vi "Begin.vi"(8 "error in":errorcluster) -> (0 "error out":errorcluster)   [LabVIEW 2019]
doc: "Called before other user functions, this VI is expected to open initial I/O refnums, load in file data, and do all program initialization. Notice that the <B>error out</B> terminal is simply used for data flow. Wiring it to other structures or subVIs ensures that this VI runs first."
uses:
  Robot Global Data.vi
  <vilib>/Rock Robotics/WPI/DriverStation/WPI_DriverStationRobotMode2.ctl
  <vilib>/Rock Robotics/WPI/Joystick/WPI_JoystickDeviceEnum.ctl
  <vilib>/Rock Robotics/Network Tables/NT Write String Array.vi
  <vilib>/Rock Robotics/WPI/ThirdParty/Phoenix-LabVIEW/Motor Controller/Controls/CTRE_Phoenix_MotorControl_NeutralMode.ctl
  <vilib>/Rock Robotics/WPI/SafetyOutput/WPI_SafetyOutputConfigMenu.ctl
  <vilib>/Rock Robotics/WPI/ThirdParty/Phoenix-LabVIEW/Motor Controller/Controls/CTRE_Phoenix_MotorControl_StatusFrameEnhanced.ctl
  <vilib>/Rock Robotics/WPI/ThirdParty/Phoenix-LabVIEW/Motor Controller/Controls/CTRE_Phoenix_MotorControl_ControlMode.ctl
  <vilib>/Rock Robotics/WPI/ThirdParty/Phoenix-LabVIEW/Motor Controller/Controls/CTRE_Phoenix_MotorControl_FeedbackDevice_TalonFX.ctl
  <vilib>/Rock Robotics/WPI/ThirdParty/Phoenix-LabVIEW/CANCoder/Controls/CTRE_Phoenix_CANcoder_SensorInitializationStrategy.ctl
  <vilib>/Rock Robotics/WPI/ThirdParty/Phoenix-LabVIEW/Motor Controller/Sensor/CTRE_Phoenix_MotorControl_SetIntegratedSensorPosition_TalonFX.vi
  <vilib>/Rock Robotics/WPI/RobotDrive/WPI_RobotDriveOpen4MotorWithExistingMotors.vi
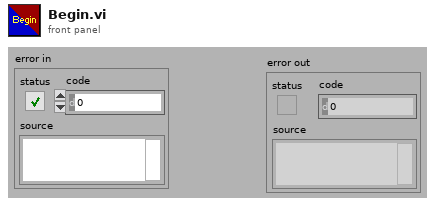
[diagram p1: front panel]
types:
  T1 = typedef "CTRE_Phoenix_MotorControl_NeutralMode.ctl" = enum8{"EEPROMSetting", "Override to Coast", "Override to Brake"}
  T2 = typedef "CTRE_Phoenix_MotorControl_ControlMode.ctl" = u16
  T3 = typedef "CTRE_Phoenix_MotorControl_StatusFrameEnhanced.ctl" = u16
  T4 = typedef "WPI_SafetyOutputConfigMenu.ctl" = enum16{"Enable", "Disable"}
  T5 = typedef "CTRE_Phoenix_CANcoder_SensorInitializationStrategy.ctl" = enum16{"Boot To Zero", "Boot To Absolute Position"}
  T6 = typedef "CTRE_Phoenix_MotorControl_FeedbackDevice_TalonFX.ctl" = i8
  T7 = typedef "WPI_JoystickDeviceEnum.ctl" = enum16{"USB 0", "USB 1", "USB 2", "USB 3", "USB 4", "USB 5"}
  T8 = typedef "WPI_DriverStationRobotMode2.ctl" = enum16{"Autonomous Disabled", "Autonomous Enabled", "Teleop Disabled", "Teleop Enabled", "Disconnected", "Finish", "Test Disabled", "Test Enabled", "Emergency Stopped"}
  T9 = typedef "WPI_JoystickDevRef.ctl" = cluster{"Device":T7}
  T10 = typedef "WPI_MotorControlDeviceRef.ctl" = cluster{"DeviceStatus":errorcluster, "Type":T11, "PWM":cluster{"PWM Channel":T12, "DeadBand":T13}, "CAN":cluster{"Device Number":u8, "SetOutput VI Ref":variant, "GetOutput VI Ref":variant, "Enable VI Ref":variant, "Disable VI Ref":variant, "Data":variant}, "Invert":bool, "DIO PWM":cluster{"PWM \"Enable\" Channel":T12, "DIOChannel":T14, "PWM Rate":dbl}}
  T11 = typedef "WPI_MotorControlType.ctl" = enum16{"PWM", "CAN", "DIO PWM"}
  T12 = typedef "FPGA_DIOPWMChannel.ctl" = enum8{"PWM 0", "PWM 1", "PWM 2", "PWM 3", "PWM 4", "PWM 5", "PWM 6", "PWM 7", "PWM 8", "PWM 9", "PWM MXP 0", "PWM MXP 1", "PWM MXP 2", "PWM MXP 3", "PWM MXP 4", "PWM MXP 5", "PWM MXP 6", "PWM MXP 7", "PWM MXP 8", "PWM MXP 9", "Invalid"}
  T13 = typedef "WPI_PWMDeadband.ctl" = cluster{"Name":string, "maxPositivePwm":i32, "minPositivePwm":i32, "centerPwm":i32, "maxNegativePwm":i32, "minNegativePwm":i32, "angularRange":u16}
  T14 = typedef "FPGA_DIOChannel.ctl" = enum8{"DIO 0", "DIO 1", "DIO 2", "DIO 3", "DIO 4", "DIO 5", "DIO 6", "DIO 7", "DIO 8", "DIO 9", "DIO MXP 0", "DIO MXP 1", "DIO MXP 2", "DIO MXP 3", "DIO MXP 4", "DIO MXP 5", "DIO MXP 6", "DIO MXP 7", "DIO MXP 8", "DIO MXP 9", "DIO MXP 10", "DIO MXP 11", "DIO MXP 12", "DIO MXP 13", "DIO MXP 14", "DIO MXP 15", "SPI Port CS1", "SPI Port CS2", "SPI Port CS3", "SPI Port MISO", "SPI Port MOSI", "Invalid"}
  T15 = typedef "WPI_RobotDriveDevRef.ctl" = cluster{"DevStatus":errorcluster, "Motors[]":T10[], "Square Inputs":bool, "Max Output":dbl}
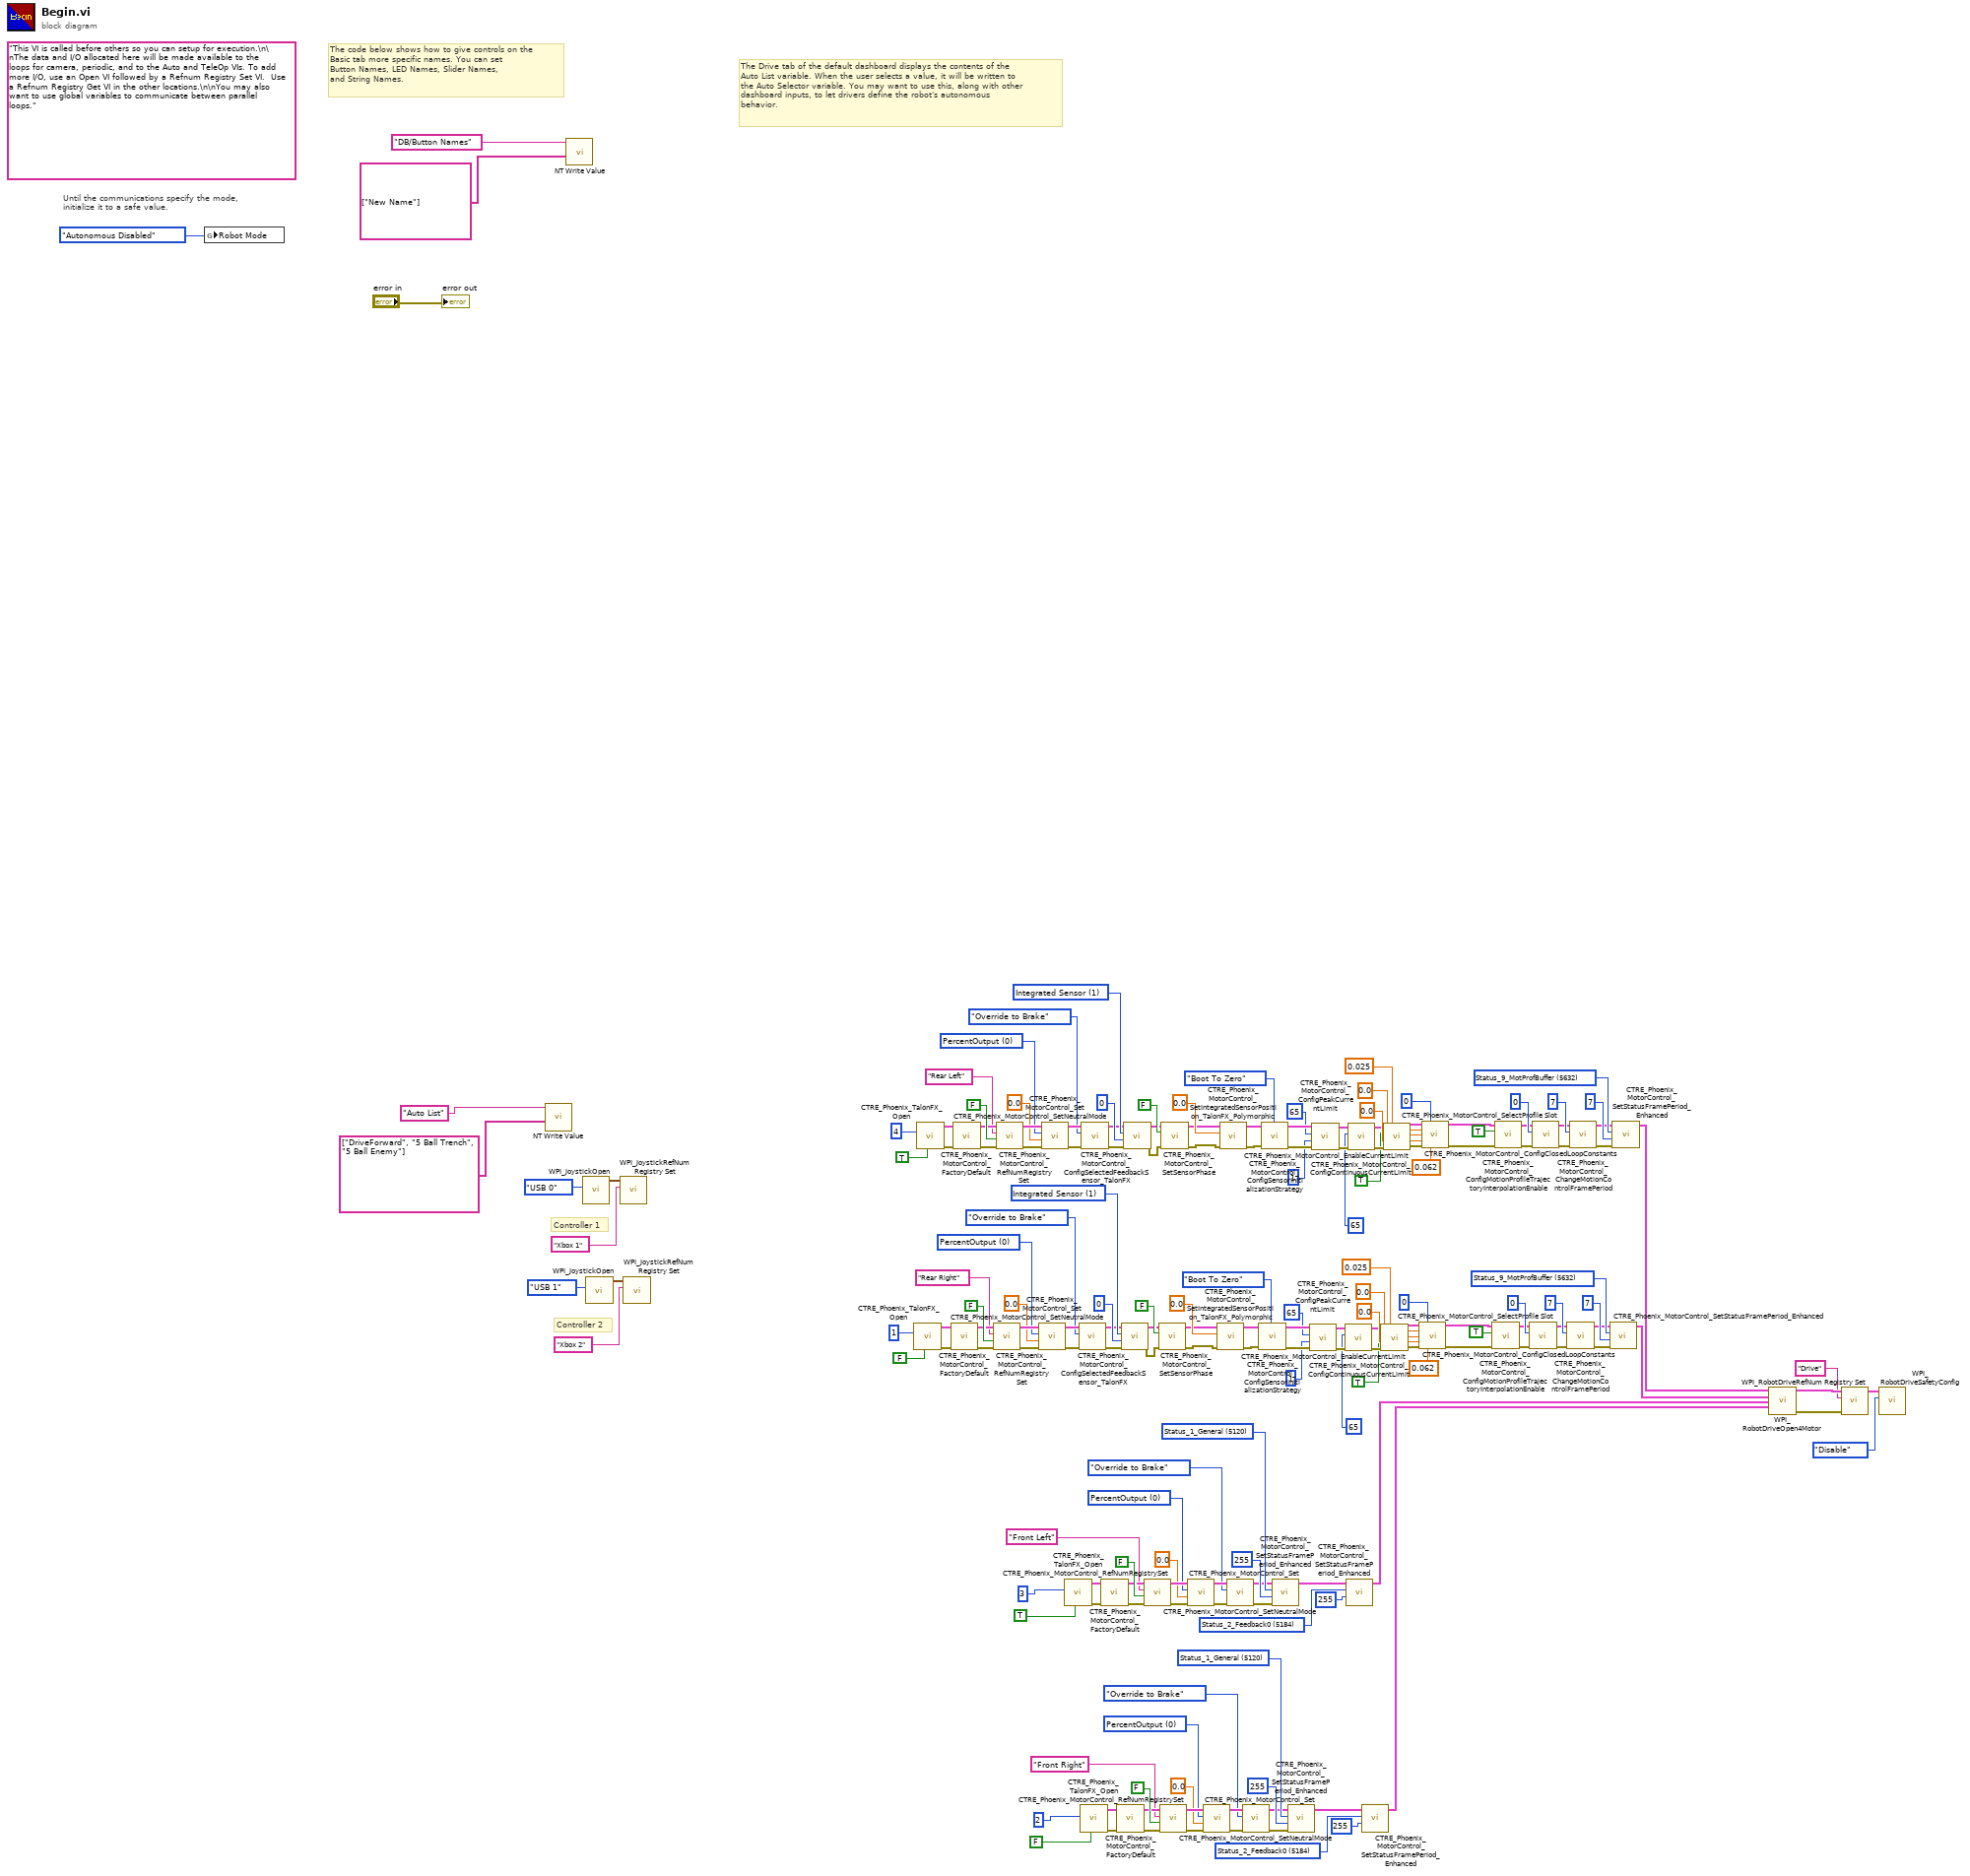
[diagram p0: block diagram]
diagram:
  w14 = T2 0 items=["PercentOutput"=0, "Position"=1, "Velocity"=2, "Current"=3, "Follower"=5, "MotionProfile"=6, "MotionMagic"=7, "MotionProfileArc"=10, "Disabled"=15] ("Control Mode")
  w21 = T3 5184 items=["Status_1_General"=5120, "Status_2_Feedback0"=5184, "Status_3_Quadrature"=5248, "Status_4_AinTempVbat"=5312, "Status_6_Misc"=5440, "Status_7_CommStatus"=5504, "Status_8_PulseWidth"=5568, "Status_9_MotProfBuffer"=5632, "Status_10_MotionMagic"=5696, "Status_11_UartGadgeteer"=5760, "Status_12_Feedback1"=5824, "Status_13_Base_PIDF0"=5888, "Status_14_Turn_PIDF1"=5952, "Status_15_FirmwareApiStatus"=6016] ("Status Frame")
  w23 = T3 5120 items=["Status_1_General"=5120, "Status_2_Feedback0"=5184, "Status_3_Quadrature"=5248, "Status_4_AinTempVbat"=5312, "Status_6_Misc"=5440, "Status_7_CommStatus"=5504, "Status_8_PulseWidth"=5568, "Status_9_MotProfBuffer"=5632, "Status_10_MotionMagic"=5696, "Status_11_UartGadgeteer"=5760, "Status_12_Feedback1"=5824, "Status_13_Base_PIDF0"=5888, "Status_14_Turn_PIDF1"=5952, "Status_15_FirmwareApiStatus"=6016] ("Status Frame")
  w37 = T2 0 items=["PercentOutput"=0, "Position"=1, "Velocity"=2, "Current"=3, "Follower"=5, "MotionProfile"=6, "MotionMagic"=7, "MotionProfileArc"=10, "Disabled"=15] ("Control Mode")
  w44 = T3 5184 items=["Status_1_General"=5120, "Status_2_Feedback0"=5184, "Status_3_Quadrature"=5248, "Status_4_AinTempVbat"=5312, "Status_6_Misc"=5440, "Status_7_CommStatus"=5504, "Status_8_PulseWidth"=5568, "Status_9_MotProfBuffer"=5632, "Status_10_MotionMagic"=5696, "Status_11_UartGadgeteer"=5760, "Status_12_Feedback1"=5824, "Status_13_Base_PIDF0"=5888, "Status_14_Turn_PIDF1"=5952, "Status_15_FirmwareApiStatus"=6016] ("Status Frame")
  w46 = T3 5120 items=["Status_1_General"=5120, "Status_2_Feedback0"=5184, "Status_3_Quadrature"=5248, "Status_4_AinTempVbat"=5312, "Status_6_Misc"=5440, "Status_7_CommStatus"=5504, "Status_8_PulseWidth"=5568, "Status_9_MotProfBuffer"=5632, "Status_10_MotionMagic"=5696, "Status_11_UartGadgeteer"=5760, "Status_12_Feedback1"=5824, "Status_13_Base_PIDF0"=5888, "Status_14_Turn_PIDF1"=5952, "Status_15_FirmwareApiStatus"=6016] ("Status Frame")
  w94 = T6 1 items=["Integrated Sensor"=1, "Sensor Sum (S0 + S1)"=9, "Sensor Difference (D0 - D1)"=10, "Remote Source 0"=11, "Remote Source 1"=12, "None"=14, "Software Emulated"=15] ("Talon FX Feedback Device")
  w96 = T2 0 items=["PercentOutput"=0, "Position"=1, "Velocity"=2, "Current"=3, "Follower"=5, "MotionProfile"=6, "MotionMagic"=7, "MotionProfileArc"=10, "Disabled"=15] ("Control Mode")
  w111 = T3 5632 items=["Status_1_General"=5120, "Status_2_Feedback0"=5184, "Status_3_Quadrature"=5248, "Status_4_AinTempVbat"=5312, "Status_6_Misc"=5440, "Status_7_CommStatus"=5504, "Status_8_PulseWidth"=5568, "Status_9_MotProfBuffer"=5632, "Status_10_MotionMagic"=5696, "Status_11_UartGadgeteer"=5760, "Status_12_Feedback1"=5824, "Status_13_Base_PIDF0"=5888, "Status_14_Turn_PIDF1"=5952, "Status_15_FirmwareApiStatus"=6016] ("Status Frame")
  w152 = T6 1 items=["Integrated Sensor"=1, "Sensor Sum (S0 + S1)"=9, "Sensor Difference (D0 - D1)"=10, "Remote Source 0"=11, "Remote Source 1"=12, "None"=14, "Software Emulated"=15] ("Talon FX Feedback Device")
  w154 = T2 0 items=["PercentOutput"=0, "Position"=1, "Velocity"=2, "Current"=3, "Follower"=5, "MotionProfile"=6, "MotionMagic"=7, "MotionProfileArc"=10, "Disabled"=15] ("Control Mode")
  w169 = T3 5632 items=["Status_1_General"=5120, "Status_2_Feedback0"=5184, "Status_3_Quadrature"=5248, "Status_4_AinTempVbat"=5312, "Status_6_Misc"=5440, "Status_7_CommStatus"=5504, "Status_8_PulseWidth"=5568, "Status_9_MotProfBuffer"=5632, "Status_10_MotionMagic"=5696, "Status_11_UartGadgeteer"=5760, "Status_12_Feedback1"=5824, "Status_13_Base_PIDF0"=5888, "Status_14_Turn_PIDF1"=5952, "Status_15_FirmwareApiStatus"=6016] ("Status Frame")
  (unwired) "This VI is called before others so you can setup for execution.\n\nThe data and I/O allocated here will be made available to the loops for camera, periodic, and to the Auto and TeleOp VIs. To add more I/O, use an Open VI followed by a Refnum Registry Set VI.  Use a Refnum Registry Get VI in the other locations.\n\nYou may also want to use global variables to communicate between parallel loops."
  # "Controller 2"
  # "Controller 1"
  # "The Drive tab of the default dashboard displays the contents of the\nAuto List variable. When the user selects a value, it will be written to\nthe Auto Selector variable. You may want to use this, along with other\ndashboard inputs, to let drivers define the robot's autonomous\nbehavior."
  # "The code below shows how to give controls on the\nBasic tab more specific names. You can set\nButton Names, LED Names, Slider Names,\nand String Names."
  # "Until the communications specify the mode,\ninitialize it to a safe value."
  n1 = global write "Robot Global Data.vi" "Robot Mode"(WPI_DriverStationRobotMode2."Autonomous Disabled" ("Robot Mode")) -> ()
  n2 = call-poly <vilib>:"NT Write Value.vi"("String Array"=string[] ["DriveForward", "5 Ball Trench", "5 Ball Enemy"], "Name"="Auto List") -> ()  [unwired: 9 in, 1 out]
  n3 = call-poly <vilib>:"NT Write Value.vi"("String Array"=string[] ["New Name"], "Name"="DB/Button Names") -> ()  [unwired: 9 in, 1 out]
  n4 = call <vilib>:"WPI_JoystickOpen.vi"("JoystickDevice"=WPI_JoystickDeviceEnum."USB 0") -> ("JoystickDevRef"=w179:T9)  [unwired: 10 in]
  n5 = call <vilib>:"WPI_JoystickOpen.vi"("JoystickDevice"=WPI_JoystickDeviceEnum."USB 1") -> ("JoystickDevRef"=w171:T9)  [unwired: 10 in]
  n6 = call <vilib>:"WPI_JoystickRefNum Registry Set.vi"("refnum name"="Xbox 1", "JoystickDevRef"=w179) -> ()  [unwired: 8 in, 2 out]
  n7 = call <vilib>:"WPI_JoystickRefNum Registry Set.vi"("refnum name"="Xbox 2", "JoystickDevRef"=w171) -> ()  [unwired: 8 in, 2 out]
  n8 = call <vilib>:"CTRE_Phoenix_TalonFX_Open.vi"("Invert"=FALSE, "Device Number"=u8 1) -> ("error out"=w79:errorcluster, "CAN Talon SRX Ref"=w81:T10)  [unwired: 8 in]
  n9 = call <vilib>:"CTRE_Phoenix_TalonFX_Open.vi"("Invert"=TRUE, "Device Number"=u8 4) -> ("error out"=w137:errorcluster, "CAN Talon SRX Ref"=w139:T10)  [unwired: 8 in]
  n10 = call <vilib>:"CTRE_Phoenix_MotorControl_FactoryDefault.vi"("error in"=w79, "PhoenixMotorControlDevRef"=w81) -> ("error out"=w78:errorcluster, "PhoenixMotorControlDevRef"=w80:T10)  [unwired: 8 in]
  n11 = call <vilib>:"CTRE_Phoenix_MotorControl_FactoryDefault.vi"("error in"=w137, "PhoenixMotorControlDevRef"=w139) -> ("error out"=w136:errorcluster, "PhoenixMotorControlDevRef"=w138:T10)  [unwired: 8 in]
  n12 = call <vilib>:"CTRE_Phoenix_MotorControl_RefNumRegistrySet.vi"("error in (no error)"=w78, "Test Mode Only"=FALSE, "refnum name"="Rear Right", "PhoenixMotorControlDevRef"=w80) -> ("error out"=w100:errorcluster, "PhoenixMotorControlDevRef"=w99:T10)  [unwired: 6 in]
  n13 = call <vilib>:"CTRE_Phoenix_MotorControl_RefNumRegistrySet.vi"("error in (no error)"=w136, "Test Mode Only"=FALSE, "refnum name"="Rear Left", "PhoenixMotorControlDevRef"=w138) -> ("error out"=w158:errorcluster, "PhoenixMotorControlDevRef"=w157:T10)  [unwired: 6 in]
  n14 = call <vilib>:"CTRE_Phoenix_MotorControl_Set.vi"("error in (no error)"=w100, "Output"=0.0, "Control Mode"=w96, "PhoenixMotorControlDevRef"=w99) -> ("error out"=w98:errorcluster, "PhoenixMotorControlDevRef"=w97:T10)  [unwired: 6 in]
  n15 = call <vilib>:"CTRE_Phoenix_MotorControl_Set.vi"("error in (no error)"=w158, "Output"=0.0, "Control Mode"=w154, "PhoenixMotorControlDevRef"=w157) -> ("error out"=w156:errorcluster, "PhoenixMotorControlDevRef"=w155:T10)  [unwired: 6 in]
  n16 = call <vilib>:"CTRE_Phoenix_TalonFX_Open.vi"("Invert"=TRUE, "Device Number"=u8 3) -> ("error out"=w32:errorcluster, "CAN Talon SRX Ref"=w34:T10)  [unwired: 8 in]
  n17 = call <vilib>:"CTRE_Phoenix_MotorControl_SetNeutralMode.vi"("error in (no error)"=w98, "Motor Control Neutral Mode"=CTRE_Phoenix_MotorControl_NeutralMode."Override to Brake", "PhoenixMotorControlDevRef"=w97) -> ("error out"=w76:errorcluster, "PhoenixMotorControlDevRef"=w77:T10)  [unwired: 7 in]
  n18 = call <vilib>:"CTRE_Phoenix_TalonFX_Open.vi"("Invert"=FALSE, "Device Number"=u8 2) -> ("error out"=w9:errorcluster, "CAN Talon SRX Ref"=w11:T10)  [unwired: 8 in]
  n19 = call <vilib>:"CTRE_Phoenix_MotorControl_SetNeutralMode.vi"("error in (no error)"=w156, "Motor Control Neutral Mode"=CTRE_Phoenix_MotorControl_NeutralMode."Override to Brake", "PhoenixMotorControlDevRef"=w155) -> ("error out"=w134:errorcluster, "PhoenixMotorControlDevRef"=w135:T10)  [unwired: 7 in]
  n20 = call <vilib>:"CTRE_Phoenix_MotorControl_FactoryDefault.vi"("error in"=w32, "PhoenixMotorControlDevRef"=w34) -> ("error out"=w31:errorcluster, "PhoenixMotorControlDevRef"=w33:T10)  [unwired: 8 in]
  n21 = call <vilib>:"CTRE_Phoenix_MotorControl_FactoryDefault.vi"("error in"=w9, "PhoenixMotorControlDevRef"=w11) -> ("error out"=w8:errorcluster, "PhoenixMotorControlDevRef"=w10:T10)  [unwired: 8 in]
  n22 = call <vilib>:"CTRE_Phoenix_MotorControl_ConfigSelectedFeedbackSensor_TalonFX.vi"("error in (no error)"=w76, "pidLoopIdx"=0, "Talon FX Feedback Device"=w94, "PhoenixMotorControlDevRef"=w77) -> ("error out"=w73:errorcluster, "PhoenixMotorControlDevRef"=w74:T10)  [unwired: 6 in]
  n23 = call <vilib>:"CTRE_Phoenix_MotorControl_ConfigSelectedFeedbackSensor_TalonFX.vi"("error in (no error)"=w134, "pidLoopIdx"=0, "Talon FX Feedback Device"=w152, "PhoenixMotorControlDevRef"=w135) -> ("error out"=w131:errorcluster, "PhoenixMotorControlDevRef"=w132:T10)  [unwired: 6 in]
  n24 = call <vilib>:"CTRE_Phoenix_MotorControl_RefNumRegistrySet.vi"("error in (no error)"=w31, "Test Mode Only"=FALSE, "refnum name"="Front Left", "PhoenixMotorControlDevRef"=w33) -> ("error out"=w41:errorcluster, "PhoenixMotorControlDevRef"=w40:T10)  [unwired: 6 in]
  n25 = call <vilib>:"CTRE_Phoenix_MotorControl_SetSensorPhase.vi"("error in (no error)"=w73, "PhaseSensor"=FALSE, "PhoenixMotorControlDevRef"=w74) -> ("error out"=w71:errorcluster, "PhoenixMotorControlDevRef"=w72:T10)  [unwired: 7 in]
  n26 = call <vilib>:"CTRE_Phoenix_MotorControl_RefNumRegistrySet.vi"("error in (no error)"=w8, "Test Mode Only"=FALSE, "refnum name"="Front Right", "PhoenixMotorControlDevRef"=w10) -> ("error out"=w18:errorcluster, "PhoenixMotorControlDevRef"=w17:T10)  [unwired: 6 in]
  n27 = call <vilib>:"CTRE_Phoenix_MotorControl_SetSensorPhase.vi"("error in (no error)"=w131, "PhaseSensor"=FALSE, "PhoenixMotorControlDevRef"=w132) -> ("error out"=w129:errorcluster, "PhoenixMotorControlDevRef"=w130:T10)  [unwired: 7 in]
  n28 = call <vilib>:"CTRE_Phoenix_MotorControl_Set.vi"("error in (no error)"=w41, "Output"=0.0, "Control Mode"=w37, "PhoenixMotorControlDevRef"=w40) -> ("error out"=w39:errorcluster, "PhoenixMotorControlDevRef"=w38:T10)  [unwired: 6 in]
  n29 = call <vilib>:"CTRE_Phoenix_MotorControl_Set.vi"("error in (no error)"=w18, "Output"=0.0, "Control Mode"=w14, "PhoenixMotorControlDevRef"=w17) -> ("error out"=w16:errorcluster, "PhoenixMotorControlDevRef"=w15:T10)  [unwired: 6 in]
  n30 = call-poly <vilib>:"CTRE_Phoenix_MotorControl_SetIntegratedSensorPosition_TalonFX_Polymorphic.vi"("error in (no error)"=w71, "New Position"=0.0, "PhoenixMotorControlDevRef"=w72) -> ("error out"=w83:errorcluster, "PhoenixMotorControlDevRef"=w82:T10)  [unwired: 7 in]
  n31 = call-poly <vilib>:"CTRE_Phoenix_MotorControl_SetIntegratedSensorPosition_TalonFX_Polymorphic.vi"("error in (no error)"=w129, "New Position"=0.0, "PhoenixMotorControlDevRef"=w130) -> ("error out"=w141:errorcluster, "PhoenixMotorControlDevRef"=w140:T10)  [unwired: 7 in]
  n32 = call <vilib>:"CTRE_Phoenix_MotorControl_SetNeutralMode.vi"("error in (no error)"=w39, "Motor Control Neutral Mode"=CTRE_Phoenix_MotorControl_NeutralMode."Override to Brake", "PhoenixMotorControlDevRef"=w38) -> ("error out"=w30:errorcluster, "PhoenixMotorControlDevRef"=w29:T10)  [unwired: 7 in]
  n33 = call <vilib>:"CTRE_Phoenix_MotorControl_SetNeutralMode.vi"("error in (no error)"=w16, "Motor Control Neutral Mode"=CTRE_Phoenix_MotorControl_NeutralMode."Override to Brake", "PhoenixMotorControlDevRef"=w15) -> ("error out"=w7:errorcluster, "PhoenixMotorControlDevRef"=w6:T10)  [unwired: 7 in]
  n34 = call <vilib>:"CTRE_Phoenix_MotorControl_ConfigSensorInitializationStrategy.vi"("error in (no error)"=w83, "Sensor Initialization Strategy"=CTRE_Phoenix_CANcoder_SensorInitializationStrategy."Boot To Zero", "PhoenixMotorControlDevRef"=w82) -> ("error out"=w63:errorcluster, "PhoenixMotorControlDevRef"=w64:T10)  [unwired: 7 in]
  n35 = call <vilib>:"CTRE_Phoenix_MotorControl_ConfigSensorInitializationStrategy.vi"("error in (no error)"=w141, "Sensor Initialization Strategy"=CTRE_Phoenix_CANcoder_SensorInitializationStrategy."Boot To Zero", "PhoenixMotorControlDevRef"=w140) -> ("error out"=w121:errorcluster, "PhoenixMotorControlDevRef"=w122:T10)  [unwired: 7 in]
  n36 = call <vilib>:"CTRE_Phoenix_MotorControl_SetStatusFramePeriod_Enhanced.vi"("error in (no error)"=w30, "periodMs"=255, "Status Frame"=w46, "PhoenixMotorControlDevRef"=w29) -> ("PhoenixMotorControlDevRef"=w42:T10)  [unwired: 6 in, 1 out]
  n37 = call <vilib>:"CTRE_Phoenix_MotorControl_SetStatusFramePeriod_Enhanced.vi"("error in (no error)"=w7, "periodMs"=255, "Status Frame"=w23, "PhoenixMotorControlDevRef"=w6) -> ("PhoenixMotorControlDevRef"=w19:T10)  [unwired: 6 in, 1 out]
  n38 = call <vilib>:"CTRE_Phoenix_MotorControl_ConfigPeakCurrentLimit.vi"("error in (no error)"=w63, "Peak Current Maximum Duration (ms)"=1, "Peak Current (Amps)"=65, "PhoenixMotorControlDevRef"=w64) -> ("error out"=w68:errorcluster, "PhoenixMotorControlDevRef"=w67:T10)  [unwired: 6 in]
  n39 = call <vilib>:"CTRE_Phoenix_MotorControl_ConfigPeakCurrentLimit.vi"("error in (no error)"=w121, "Peak Current Maximum Duration (ms)"=1, "Peak Current (Amps)"=65, "PhoenixMotorControlDevRef"=w122) -> ("error out"=w126:errorcluster, "PhoenixMotorControlDevRef"=w125:T10)  [unwired: 6 in]
  n40 = call <vilib>:"CTRE_Phoenix_MotorControl_ConfigContinuousCurrentLimit.vi"("error in (no error)"=w68, "Continuous Current Limit (Amps)"=65, "PhoenixMotorControlDevRef"=w67) -> ("error out"=w66:errorcluster, "PhoenixMotorControlDevRef"=w65:T10)  [unwired: 7 in]
  n41 = call <vilib>:"CTRE_Phoenix_MotorControl_SetStatusFramePeriod_Enhanced.vi"("periodMs"=255, "Status Frame"=w44, "PhoenixMotorControlDevRef"=w42) -> ("PhoenixMotorControlDevRef"=w24:T10)  [unwired: 7 in, 1 out]
  n42 = call <vilib>:"CTRE_Phoenix_MotorControl_ConfigContinuousCurrentLimit.vi"("error in (no error)"=w126, "Continuous Current Limit (Amps)"=65, "PhoenixMotorControlDevRef"=w125) -> ("error out"=w124:errorcluster, "PhoenixMotorControlDevRef"=w123:T10)  [unwired: 7 in]
  n43 = call <vilib>:"CTRE_Phoenix_MotorControl_SetStatusFramePeriod_Enhanced.vi"("periodMs"=255, "Status Frame"=w21, "PhoenixMotorControlDevRef"=w19) -> ("PhoenixMotorControlDevRef"=w1:T10)  [unwired: 7 in, 1 out]
  n44 = call <vilib>:"CTRE_Phoenix_MotorControl_EnableCurrentLimit.vi"("error in (no error)"=w66, "Enable Current Limit?"=TRUE, "PhoenixMotorControlDevRef"=w65) -> ("error out"=w61:errorcluster, "PhoenixMotorControlDevRef"=w62:T10)  [unwired: 7 in]
  n45 = call <vilib>:"CTRE_Phoenix_MotorControl_EnableCurrentLimit.vi"("error in (no error)"=w124, "Enable Current Limit?"=TRUE, "PhoenixMotorControlDevRef"=w123) -> ("error out"=w119:errorcluster, "PhoenixMotorControlDevRef"=w120:T10)  [unwired: 7 in]
  n46 = call <vilib>:"CTRE_Phoenix_MotorControl_ConfigClosedLoopConstants.vi"("PhoenixMotorControlDevRef"=w62, "slotIdx"=0, "P"=0.025, "I"=0.0, "D"=0.0, "error in (no error)"=w61, "F"=0.062) -> ("PhoenixMotorControlDevRef"=w70:T10, "error out"=w69:errorcluster)  [unwired: 7 in]
  n47 = call <vilib>:"CTRE_Phoenix_MotorControl_ConfigClosedLoopConstants.vi"("PhoenixMotorControlDevRef"=w120, "slotIdx"=0, "P"=0.025, "I"=0.0, "D"=0.0, "error in (no error)"=w119, "F"=0.062) -> ("PhoenixMotorControlDevRef"=w128:T10, "error out"=w127:errorcluster)  [unwired: 7 in]
  n48 = call <vilib>:"CTRE_Phoenix_MotorControl_ConfigMotionProfileTrajectoryInterpolationEnable.vi"("error in"=w69, "enable?"=TRUE ("PhaseSensor"), "PhoenixMotorControlDevRef"=w70) -> ("error out"=w104:errorcluster, "PhoenixMotorControlDevRef"=w101:T10)  [unwired: 7 in]
  n49 = call <vilib>:"CTRE_Phoenix_MotorControl_ConfigMotionProfileTrajectoryInterpolationEnable.vi"("error in"=w127, "enable?"=TRUE ("PhaseSensor"), "PhoenixMotorControlDevRef"=w128) -> ("error out"=w162:errorcluster, "PhoenixMotorControlDevRef"=w159:T10)  [unwired: 7 in]
  n50 = call <vilib>:"CTRE_Phoenix_MotorControl_SelectProfile Slot.vi"("error in (no error)"=w104, "slotIdx"=0, "PhoenixMotorControlDevRef"=w101) -> ("error out"=w103:errorcluster, "PhoenixMotorControlDevRef"=w107:T10)  [unwired: 7 in]
  n51 = call <vilib>:"CTRE_Phoenix_MotorControl_SelectProfile Slot.vi"("error in (no error)"=w162, "slotIdx"=0, "PhoenixMotorControlDevRef"=w159) -> ("error out"=w161:errorcluster, "PhoenixMotorControlDevRef"=w165:T10)  [unwired: 7 in]
  n52 = call <vilib>:"CTRE_Phoenix_MotorControl_ChangeMotionControlFramePeriod.vi"("error in"=w103, "periodMs"=7, "PhoenixMotorControlDevRef"=w107) -> ("error out"=w102:errorcluster, "PhoenixMotorControlDevRef"=w109:T10)  [unwired: 7 in]
  n53 = call <vilib>:"CTRE_Phoenix_MotorControl_ChangeMotionControlFramePeriod.vi"("error in"=w161, "periodMs"=7, "PhoenixMotorControlDevRef"=w165) -> ("error out"=w160:errorcluster, "PhoenixMotorControlDevRef"=w167:T10)  [unwired: 7 in]
  n54 = call <vilib>:"CTRE_Phoenix_MotorControl_SetStatusFramePeriod_Enhanced.vi"("error in (no error)"=w102, "periodMs"=7, "Status Frame"=w111, "PhoenixMotorControlDevRef"=w109) -> ("PhoenixMotorControlDevRef"=w47:T10)  [unwired: 6 in, 1 out]
  n55 = call <vilib>:"CTRE_Phoenix_MotorControl_SetStatusFramePeriod_Enhanced.vi"("error in (no error)"=w160, "periodMs"=7, "Status Frame"=w169, "PhoenixMotorControlDevRef"=w167) -> ("PhoenixMotorControlDevRef"=w48:T10)  [unwired: 6 in, 1 out]
  n56 = call-poly <vilib>:"WPI_RobotDriveOpen4Motor.vi"("Rear Left Motor Dev Ref"=w48, "Rear Right Motor Dev Ref"=w47, "Front Left Motor Dev Ref"=w24, "Front Right Motor Dev Ref"=w1) -> ("RobotDriveDevRef"=w53:T15, "error out"=w51:errorcluster)  [unwired: 10 in]
  n57 = call <vilib>:"WPI_RobotDriveRefNum Registry Set.vi"("error in (no error)"=w51, "refnum name"="Drive", "RobotDriveDevRef"=w53) -> ("RobotDriveDevRef"=w50:T15)  [unwired: 1 in, 7 out]
  n58 = call <vilib>:"WPI_RobotDriveSafetyConfig.vi"("mode"=WPI_SafetyOutputConfigMenu."Disable", "RobotDriveDevRef"=w50) -> ()  [unwired: 8 in, 2 out]
  "error out" <- "error in"
